vi "Read TemporalData.vi"(8 "error in (no error)":errorcluster, 10 "ReadSize":u32, 11 "AODAcq in":refnum<class "AODAcq.lvclass">) -> (0 "error out":errorcluster, 2 "TemporalData":waveform(i32)[](array[waveform]), 3 "AODAcq out":refnum<class "AODAcq.lvclass">)   [LabVIEW 2011, in "AODAcq.lvclass"]
uses:
  AODAcq.lvclass
  AODAcq.lvclass/AODAcq.ctl
  <vilib>/Utility/error.llb/Error Cluster From Error Code.vi
  <vilib>/rvi/errors/niLvFpgaAdjustHostInterfaceError.vi
  HDF5Tools/LabView/Append To Dataset 2D Double.vi
  <vilib>/rvi/interface/nirviMethod/nirviMethod.xnode
  FPGA_Control/AODRef.ctl
  FPGA Bitfiles/Acquisition_FPGATarget_AODControl(FPGA)_C1C38267.lvbitx
  FPGA_Control/AOD Control (FPGA).vi
  HDF5Tools/LabView/HDF5Tools.lvlib
  <vilib>/FPGAPlugInAG/PXIe-7965R/niLvFpga_ReadFifo_PXIe-7965R.vi
  <vilib>/rvi/errors/niLvFpgaMergeErrorWithErrorCode.vi
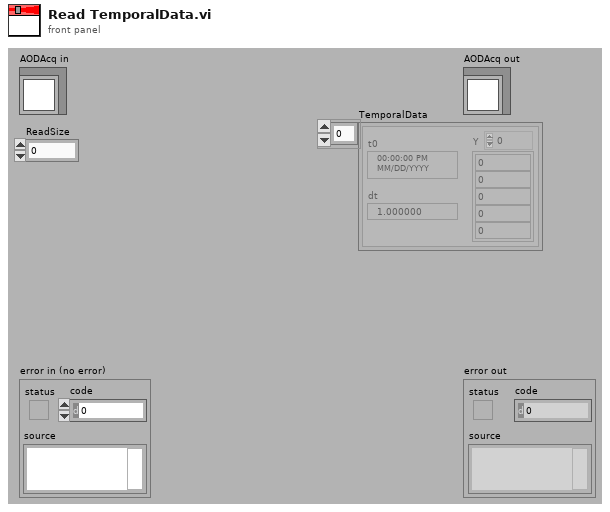
[diagram p1: front panel]
types:
  T1 = typedef "AODRef.ctl" = refnum<k20>
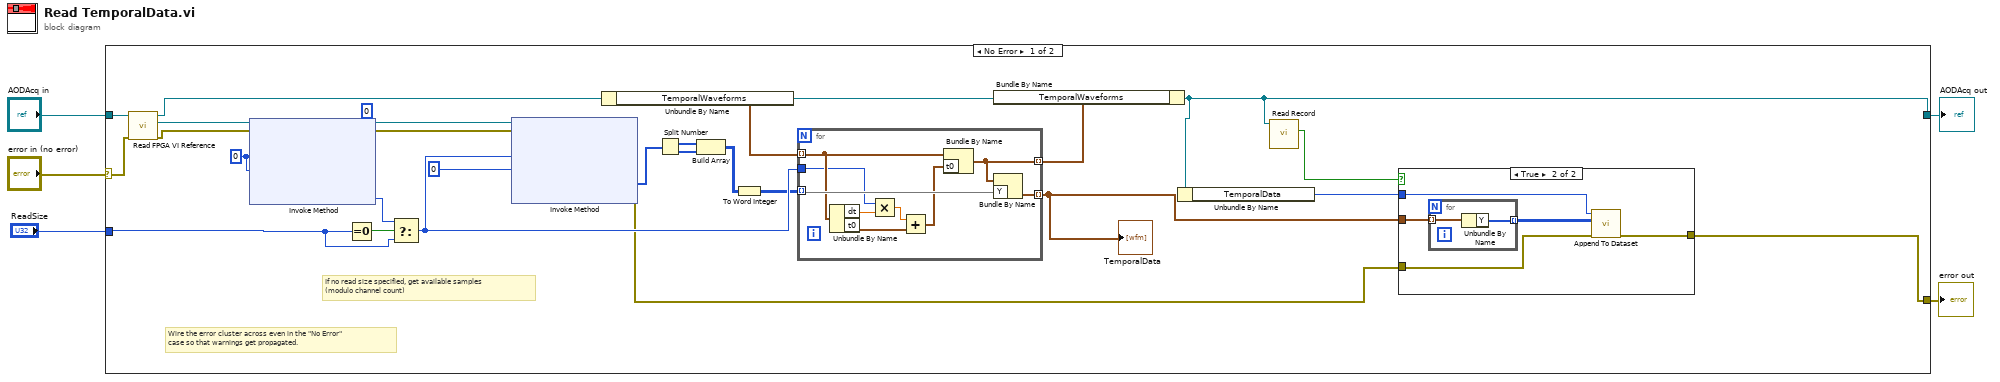
[diagram p0: block diagram]
diagram:
  n1 = case shown="No Error" "error in (no error)" {
    selector: "error in (no error)" -> [w25 w50]
    tunnel: [w7 w50] -> w4
    tunnel: [w9 w49] -> w2
    tunnel: "AODAcq in" -> [w31 w49]
    tunnel: "ReadSize" -> [w21 _]
    frame No Error {
      (unwired) u32 0 ("y")
      w30 = u32 0 ("Number of Elements")
      # "If no read size specified, get available samples \n(modulo channel count)"
      # "Wire the error cluster across even in the \"No Error\"\ncase so that warnings get propagated."
      n2 = call-dynamic "Read FPGA VI Reference.vi"("error in (no error)"=w25, "AODAcq in"=w31) -> ("error out"=w13:errorcluster, "FPGA VI Reference"=w14:T1, "AODAcq out"=w23:refnum<class "AODAcq.lvclass">)  [unwired: 7 in]
      n3 = xnode "Invoke Method"("FPGA VI Reference In"=w14, "error in"=w13, "Number of Elements"=w30, "Timeout (ms)"=w30) -> ("FPGA VI Reference Out"=w28:T1, "error out"=w27:errorcluster, "Elements Remaining"=w20:u32)  [unwired: 1 out]
      n4 = Equal To 0?(x=w21) -> (x = 0?=w29:bool)
      n5 = Select(t=w20, s=w29, f=w21) -> (s? t:f=w15:u32)
      n6 = xnode "Invoke Method"("FPGA VI Reference In"=w28, "error in"=w27, "Number of Elements"=w15, "Timeout (ms)"=0) -> ("error out"=w8:errorcluster, "Data"=w19:i32[])  [unwired: 2 out]
      n7 = Unbundle By Name(w23) -> ("TemporalWaveforms"=w24:waveform(i32)[])
      n8 = Split Number(x=w19) -> (hi(x)=w17:u16[], lo(x)=w18:u16[])
      n9 = Build Array(w17, w18) -> (w16:u16[][])
      n10 = To Word Integer(number=w16) -> (16bit integer=w12:i16[][])
      n11 = for {
        tunnel: w12 -> [w48] mode=indexing
        tunnel: [w47] -> w6 mode=indexing
        tunnel: w24 -> [w43] mode=indexing
        tunnel: w15 -> [w40]
        tunnel: [w41] -> w22 mode=indexing
        n12 = Unbundle By Name(w43) -> ("dt"=w46:dbl, "t0"=w44:timestamp)
        n13 = Multiply(x=w40, y=w46) -> (x*y=w45:dbl)
        n14 = Add(x=w45, y=w44) -> (x+y=w42:timestamp)
        n15 = Bundle By Name(cluster=w43, "t0"=w42) -> (w41:waveform(i32))
        n16 = Bundle By Name(cluster=w41, "Y"=w48) -> (w47:waveform(i32))
      }
      "TemporalData" <- w6
      n17 = Bundle By Name(cluster=w23, "TemporalWaveforms"=w22) -> (w9:refnum<class "AODAcq.lvclass">)
      n18 = Unbundle By Name(w9) -> ("TemporalData"=w11:i32)
      n19 = call-dynamic "Read Record.vi"("AODAcq in"=w9) -> ("Record"=w10:bool)  [unwired: 8 in, 2 out]
      n20 = case shown="True" w10 {
        tunnel: w6 -> [_ w37]
        tunnel: w11 -> [_ w34]
        tunnel: w8 -> [w32 w35]
        tunnel: [w32 w33] -> w7
        frame False {
        }
        frame True {
          n21 = for {
            tunnel: w37 -> [w39] mode=indexing
            tunnel: [w38] -> w36 mode=indexing
            n22 = Unbundle By Name(w39) -> ("Y"=w38:i32[])
          }
          n23 = call-poly "Append To Dataset.vi"("Error in (no error)"=w35, "Data"=w36, "Dataset id in"=w34) -> ("Error out"=w33:errorcluster)  [unwired: 7 in, 1 out]
        }
      }
    }
    frame Error {
    }
  }
  "error out" <- w4
  "AODAcq out" <- w2
